vi "Lvi Read Dbl Data1D.vi"(7 "OnlyReadAvailable":bool, 8 "error in (no error)":errorcluster, 9 "timeout":dbl, 10 "TaskRef":i32, 11 "DataBufSize":u32) -> (0 "error out":errorcluster, 1 "DataBuf":dbl[](array[numeric]), 2 "TaskRef out":i32, 3 "DataBufSize out":u32, 5 "function return":u32(ring))   [LabVIEW 2022 SP3, in "DtLvLink.lvlib"]
doc: "Calls directly into the entry points of the DLL of the Data Acq SDK to return a one-dimensional array of double data points from the specified task. This VI is used by the higher-level VI, DtOLRead."
uses:
  DtLvLink.lvlib
  <userlib>/LV-Link3/DtLvLink_64.dll
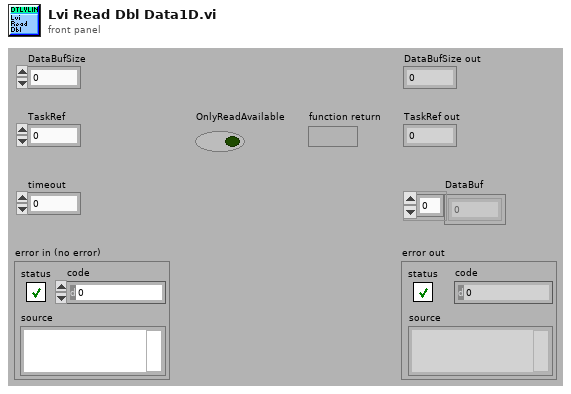
[diagram p1: front panel]
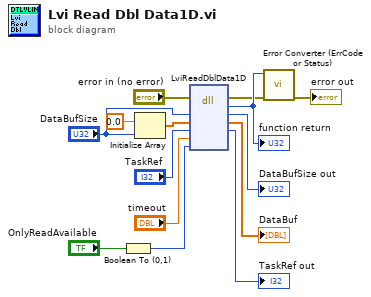
[diagram p0: block diagram]
diagram:
  n1 = Boolean To (0,1)(Boolean="OnlyReadAvailable") -> (0, 1=w4:i16)
  n2 = Initialize Array(0.0 ("element"), "DataBufSize") -> (w11:dbl[])
  n3 = dll-call lib="C:/Program Files/National Instruments/LabVIEW 2022/user.lib/LV-Link3/DtLvLink_64.*" fn="LviReadDblData1D"(error in="error in (no error)", "DataBufSize"="DataBufSize", "DataBuf"=w11, "TaskRef"="TaskRef", "timeout"="timeout", "OnlyReadAvailable"=w4) -> (error out=w2:errorcluster, w14:u32, "DataBufSize"=→"DataBufSize out":u32, "DataBuf"=→"DataBuf":dbl[], "TaskRef"=→"TaskRef out":i32)  [unwired: 4 in, 1 out]
  "function return" <- w14
  n4 = call "Error Converter (ErrCode or Status).vi"("error in (no error)"=w2, "error code"=w14) -> ("error out"=→"error out":errorcluster)  [unwired: 9 in]
